vi "DEM.vi"(0 "System no.":i32=1 min=1 max=4 step=1, 5 "error in":errorcluster) -> (19 "error out":errorcluster)   [LabVIEW 2020]
doc: "Starts demo mode of the system controller. Use #24 to stop demo."
panel:
  # "Starts demo mode of the system controller, use #24.vi to stop demo."
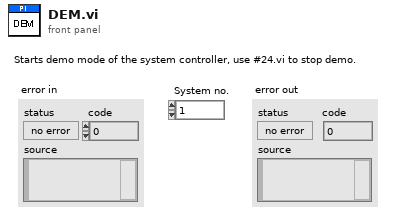
[diagram p1: front panel]
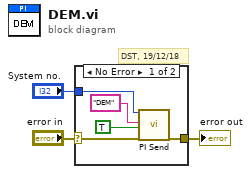
[diagram p0: block diagram]
diagram:
  # "DST, 19/12/18"
  n1 = case shown="No Error" "error in" {
    selector: "error in" -> [w4 w9]
    tunnel: "System no." -> [w6 _]
    tunnel: [w5 w9] -> w2
    frame No Error {
      n2 = call "PI Send.vi"("System no."=w6, "String to send"="DEM", "Attach termination char.?"=TRUE ("Attach Linefeed?"), "error in"=w4) -> ("error out"=w5:errorcluster)  [unwired: 2 in, 13 out]
    }
    frame Error {
    }
  }
  "error out" <- w2
